vi "Connect.vi"(8 "error in (no error)":errorcluster, 9 "IP Address/USB":string="192.109.209.128", 10 "Timeout (5s)":u8=5, 11 ".dll Path":path) -> (0 "error out":errorcluster, 3 "Potentiostat Galvanostat out":refnum<class "Potentiostat Galvanostat.lvclass">)   [LabVIEW 2018, in "Potentiostat Galvanostat.lvclass"]
uses:
  Potentiostat Galvanostat.lvclass
  Potentiostat Galvanostat.lvclass/Potentiostat Galvanostat.ctl
  BL_GetErrorMsg.vi
  <vilib>/Utility/error.llb/Error Cluster From Error Code.vi
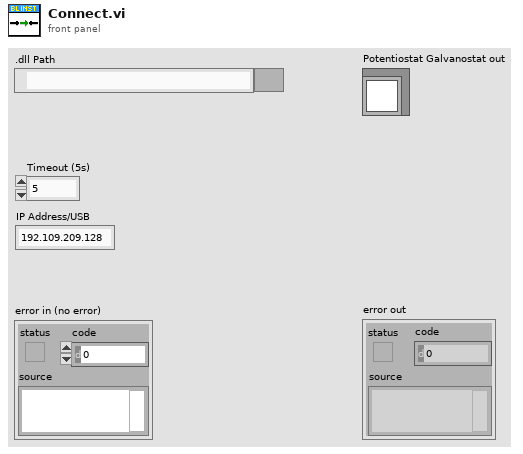
[diagram p1: front panel]
types:
  T1 = typedef "Potentiostat Galvanostat.lvclass/Device Information.ctl" = cluster{"Device Code":T2, "RAM Size":i32, "CPU":i32, "Number Of Channels":i32, "Number Of Slots":i32, "Firmware Version":i32, "Firmware Year":i32, "Firmware Month":i32, "Firmware Day":i32, "HT Display On":i32, "No. of Connected PCs":i32}
  T2 = typedef "Potentiostat Galvanostat.lvclass/Device Code.ctl" = i32
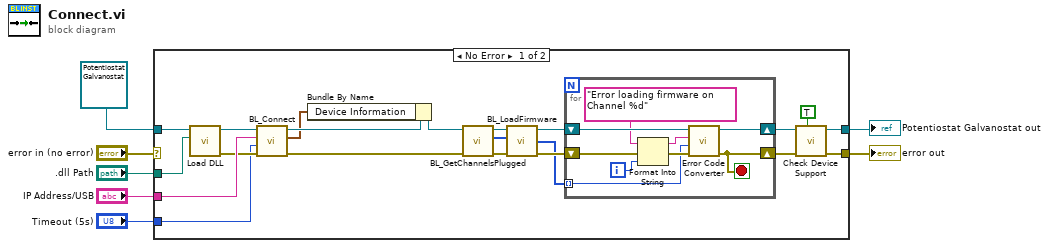
[diagram p0: block diagram]
diagram:
  n1 = case shown="No Error" "error in (no error)" {
    selector: "error in (no error)" -> [_ w39]
    tunnel: [w14 w39] -> w6
    tunnel: [w12 w38] -> w2
    tunnel: refnum<class "Potentiostat Galvanostat.lvclass"> refnum ("Potentiostat Galvanostat in") -> [w28 w38]
    tunnel: ".dll Path" -> [w27 _]
    tunnel: "IP Address/USB" -> [w26 _]
    tunnel: "Timeout (5s)" -> [w13 _]
    frame No Error {
      n2 = call "Load DLL.vi"("DLL Path"=w27, "Potentiostat Galvanostat in"=w28) -> ("error out"=w25:errorcluster, "Potentiostat Galvanostat out"=w24:refnum<class "Potentiostat Galvanostat.lvclass">)  [unwired: 8 in]
      n3 = call "BL_Connect.vi"("error in (no error)"=w25, "Timeout"=w13, "IP Address"=w26, "Potentiostat Galvanostat in"=w24) -> ("error out"=w23:errorcluster, "Device Information"=w8:T1, "Potentiostat Galvanostat out"=w10:refnum<class "Potentiostat Galvanostat.lvclass">)  [unwired: 5 in]
      n4 = Bundle By Name(cluster=w10, "Device Information"=w8) -> (w9:refnum<class "Potentiostat Galvanostat.lvclass">)
      n5 = call-dynamic "BL_GetChannelsPlugged .vi"("error in (no error)"=w23, "Potentiostat Galvanostat in"=w9) -> ("error out"=w22:errorcluster, "Plugged Channels"=w20:u8[], "Potentiostat Galvanostat out"=w21:refnum<class "Potentiostat Galvanostat.lvclass">)  [unwired: 7 in]
      n6 = call "BL_LoadFirmware.vi"("Potentiostat Galvanostat in"=w21, "Channels"=w20, "error in (no error)"=w22) -> ("Potentiostat Galvanostat out"=w17:refnum<class "Potentiostat Galvanostat.lvclass">, "Channel Error Codes"=w18:i32[], "error out"=w19:errorcluster)  [unwired: 9 in, 1 out]
      n7 = for {
        tunnel: w18 -> [w29] mode=indexing
        shift-right: [w36] -> w15
        shift-left: w17 -> [w37]
        shift-right: [w35] -> w16
        shift-left: w19 -> [w34]
        i -> [w32]
        stop <- w35 stop-if-true
        n8 = Format Into String(initial string="Error loading firmware on Channel %d", error in=w34, w32) -> (resulting string=w30:string, error out=w33:errorcluster)  [unwired: 1 in]
        n9 = call "Error Code Converter.vi"("error in (no error)"=w33, "Error Code"=w29, "Additional Description"=w30, "Potentiostat Galvanostat in"=w37) -> ("error out"=w35:errorcluster, "Potentiostat Galvanostat out"=w36:refnum<class "Potentiostat Galvanostat.lvclass">)  [unwired: 6 in]
      }
      n10 = call "Check Device Support.vi"("Output Error?"=TRUE, "error in (no error)"=w16, "Potentiostat Galvanostat in"=w15) -> ("error out"=w14:errorcluster, "Potentiostat Galvanostat out"=w12:refnum<class "Potentiostat Galvanostat.lvclass">)  [unwired: 6 in, 1 out]
    }
    frame Error {
    }
  }
  "error out" <- w6
  "Potentiostat Galvanostat out" <- w2
